vi "gun_speed_control.vi"(9 "Period (sec)":dbl, 10 "Speed (rps)":dbl, 11 "Gun Const":T1={"gun"={"num_lines"=0.0, "gain_kp1"=0.0, "gain_kp2"=0.0, "gain_ki"=0.0, "gain_kd"=0.0}, "turret"={"center_ana"=0.0, "volts_per_180"=0.0, "man_scale"=0.0, "turret_idg"={"low_fault_ana"=0.0, "high_fault_ana"=0.0, "min_ana"=0.0, "max_ana"=0.0, "movement_thresh"=0.0, "movement_time"=0.0}, "turret_pid"={"kP"=0.0, "kI"=0.0, "kD"=0.0}, "turret_invert"=TRUE, "turret_low_power"=0.0}, "tracking"={"velocity_lead_gain"=0.0, "velocity_rotation_gain"=0.0}, "hood"={"hood_idg"={"low_fault_ana"=0.0, "high_fault_ana"=0.0, "min_ana"=0.0, "max_ana"=0.0, "movement_thresh"=0.0, "movement_time"=0.0}, "hood_pid"={"kP"=0.0, "kI"=0.0, "kD"=0.0}, "hood_scale"={"min_ana"=0.0, "min_units"=0.0, "max_ana"=0.0, "max_units"=0.0}, "hood_invert"=FALSE}}) -> (1 "rpm raw":dbl, 2 "Sensor Speed (rps)":dbl, 3 "Output":dbl)   [LabVIEW 2011]
uses:
  gun_const_t.ctl
  gun_idg_const.ctl
  common/gain_const.ctl
  common/scale_const.ctl
  signals/Signal.ctl
  <vilib>/ptbypt/NI_PtbyPt.lvlib
  <vilib>/Analysis/3filter.llb/Filter Passband Type.ctl
  <vilib>/Analysis/NI_AALBase.lvlib
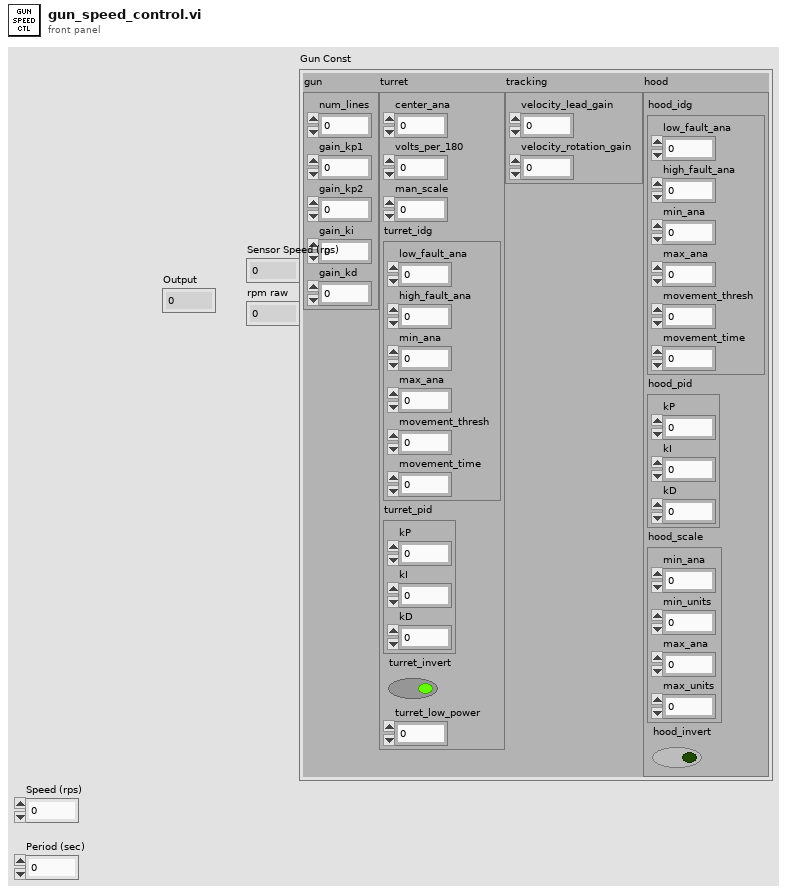
[diagram p1: front panel]
types:
  T1 = typedef "gun_const_t.ctl" = cluster{"gun":cluster{"num_lines":dbl, "gain_kp1":dbl, "gain_kp2":dbl, "gain_ki":dbl, "gain_kd":dbl}, "turret":cluster{"center_ana":dbl, "volts_per_180":dbl, "man_scale":dbl, "turret_idg":T2, "turret_pid":T3, "turret_invert":bool, "turret_low_power":dbl}, "tracking":cluster{"velocity_lead_gain":dbl, "velocity_rotation_gain":dbl}, "hood":cluster{"hood_idg":T2, "hood_pid":T3, "hood_scale":T4, "hood_invert":bool}}
  T2 = typedef "gun_idg_const.ctl" = cluster{"low_fault_ana":dbl, "high_fault_ana":dbl, "min_ana":dbl, "max_ana":dbl, "movement_thresh":dbl, "movement_time":dbl}
  T3 = typedef "gain_const.ctl" = cluster{"kP":dbl, "kI":dbl, "kD":dbl}
  T4 = typedef "scale_const.ctl" = cluster{"min_ana":dbl, "min_units":dbl, "max_ana":dbl, "max_units":dbl}
  T5 = typedef "Signal.ctl" = enum16{"SIGFIRE", "SIGSTOPSCRIPT", "SIGSTARTGUN", "SIGSTOPGUN", "SIGDISABLED", "SIGENABLED", "SIGUDPTIMEOUT", "SIGNEWVISION_REMOTE", "SIGNEWVISION_LOCAL"}
  T6 = typedef "NI_AALBase.lvlib/Filter Passband Type.ctl" = enum32{"Lowpass", "Highpass", "Bandpass", "Bandstop"}
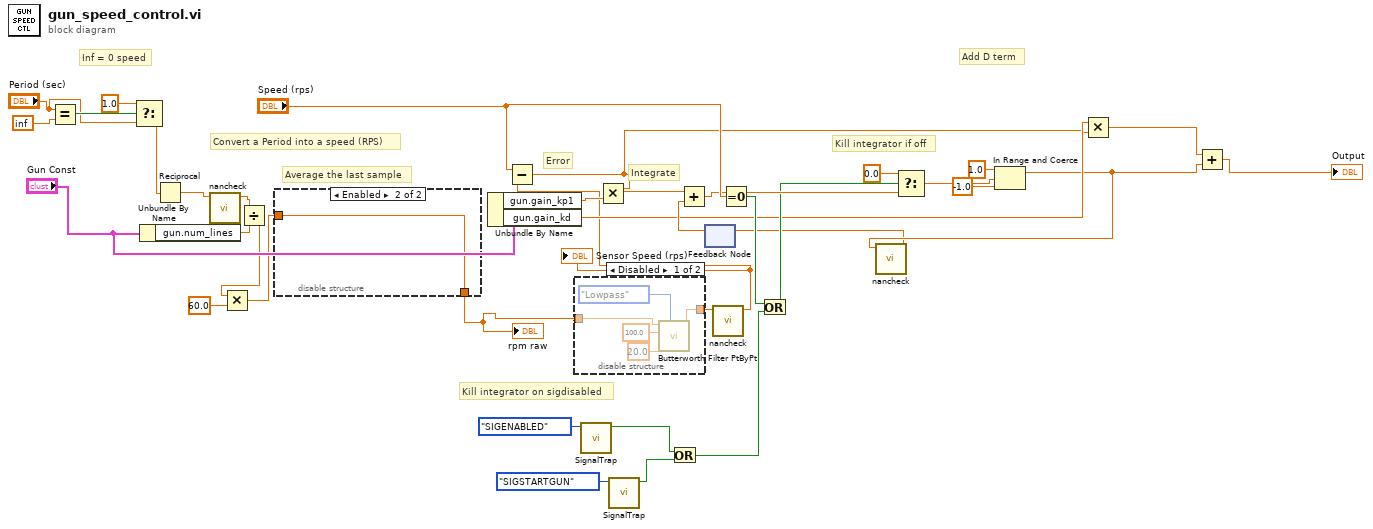
[diagram p0: block diagram]
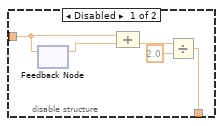
[diagram p3: hidden frame]
diagram:
  # "Add D term"
  # "Inf = 0 speed"
  # "Kill integrator on sigdisabled"
  # "Average the last sample"
  # "Kill integrator if off"
  # "Integrate"
  # "Error"
  # "Convert a Period into a speed (RPS)"
  n1 = Equal?(x="Period (sec)", y=inf) -> (x = y?=w22:bool)
  n2 = Select(t=1.0, s=w22, f="Period (sec)") -> (s? t:f=w9:dbl)
  n3 = Unbundle By Name("Gun Const") -> ("gun.num_lines"=w36:dbl)
  n4 = Reciprocal(x=w9) -> (1/x=w10:dbl)
  n5 = call "nancheck.vi"("nancheck_in"=w10) -> ("nancheck_out"=w11:dbl)  [unwired: 10 in]
  n6 = Divide(x=w11, y=w36) -> (x/y=w2:dbl)
  n7 = Multiply(x=w2, y=60.0) -> (x*y=w3:dbl)
  n8 = disable-structure shown="Enabled" {
    disable-tunnel: w3 -> [w39 w43]
    disable-tunnel: [w38 w43] -> w4
    frame Disabled {
      n9 = feedback #1() -> (w40:dbl)  [unwired: 1 in]
      n10 = feedback-in #1(w39) -> ()
      n11 = Compound Arithmetic op=ADD(w39, w40) -> (w41:dbl)
      n12 = Divide(x=w41, y=2.0) -> (x/y=w38:dbl)
    }
    frame Enabled {
    }
  }
  "rpm raw" <- w4
  n13 = Unbundle By Name("Gun Const") -> ("gun.gain_kp1"=w37:dbl, "gun.gain_kd"=w17:dbl)
  n14 = disable-structure shown="Disabled" {
    disable-tunnel: w4 -> [w45 w49]
    disable-tunnel: [w44 w49] -> w12
    frame Disabled {
      n15 = call <vilib>:"Butterworth Filter PtByPt.vi"("filter type"=Filter_Passband_Type."Lowpass", "low cutoff freq: fl"=20.0, "sampling freq: fs"=100.0, "x"=w45) -> ("Filtered x"=w44:dbl)  [unwired: 5 in, 1 out]
    }
    frame Enabled {
    }
  }
  n16 = call "SignalTrap.vi"("Signal"=Signal."SIGENABLED") -> ("Trapped Signal"=w7:bool)  [unwired: 10 in]
  n17 = call "SignalTrap.vi"("Signal"=Signal."SIGSTARTGUN") -> ("Trapped Signal"=w6:bool)  [unwired: 10 in]
  n18 = Or(x=w7, y=w6) -> (x .or. y?=w5:bool)
  n19 = feedback #2() -> (w32:dbl)  [unwired: 1 in]
  n20 = call "nancheck.vi"("nancheck_in"=w12) -> ("nancheck_out"=w13:dbl)  [unwired: 10 in]
  "Sensor Speed (rps)" <- w13
  n21 = Subtract(x="Speed (rps)", y=w13) -> (x-y=w16:dbl)
  n22 = Multiply(x=w16, y=w37) -> (x*y=w31:dbl)
  n23 = Add(x=w31, y=w32) -> (x+y=w33:dbl)
  n24 = Equal To 0?(x="Speed (rps)") -> (x = 0?=w25:bool)
  n25 = Or(x=w25, y=w5) -> (x .or. y?=w24:bool)
  n26 = Select(t=0.0, s=w24, f=w33) -> (s? t:f=w29:dbl)
  n27 = In Range and Coerce(upper limit=1.0, x=w29, lower limit=-1.0) -> (coerced(x)=w15:dbl)  [unwired: 1 out]
  n28 = call "nancheck.vi"("nancheck_in"=w15) -> ("nancheck_out"=w14:dbl)  [unwired: 10 in]
  n29 = feedback-in #2(w14) -> ()
  n30 = Multiply(x=w17, y=w16) -> (x*y=w18:dbl)
  n31 = Add(x=w18, y=w15) -> (x+y=→"Output":dbl)
